vi "Create Sections from Path.vi"(8 "error in":errorcluster, 10 "Path":string, 11 "Device BaseNodeType in":T1) -> (0 "error out":errorcluster, 1 "SectionRef":T1, 2 "NewRef?":bool, 3 "Device BaseNodeType out":T1, 4 "ChannelName":string)   [LabVIEW 2010, in "RefMem PtByPt Custom Device.lvlib"]
uses:
  Custom Device/RefMem PtByPt Custom Device.lvlib
  <vilib>/NI Veristand/Custom Device API/Custom Device Pointer.ctl
  NationalInstruments.VeriStand.SystemStorage
  Custom Device/Controls/Global.vi
  <vilib>/NI Veristand/Custom Device API/Custom Device API.lvlib
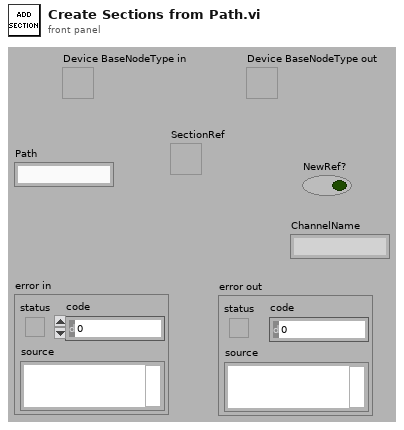
[diagram p1: front panel]
types:
  T1 = typedef "Custom Device API.lvlib/Custom Device Pointer.ctl" = refnum<k24>
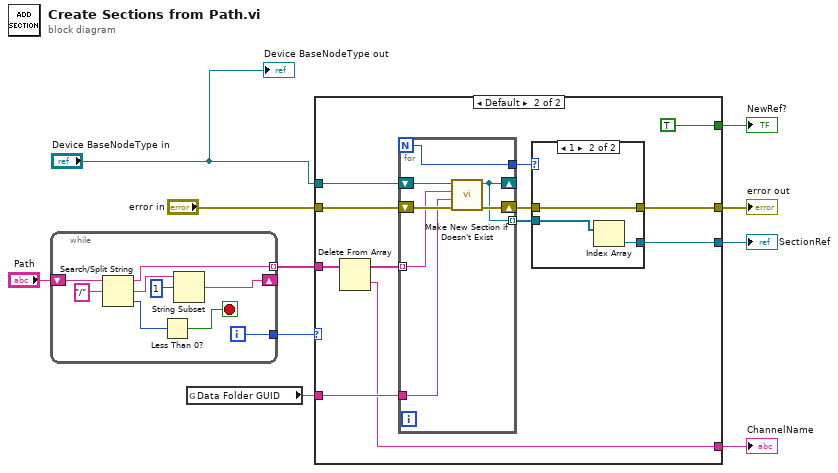
[diagram p0: block diagram]
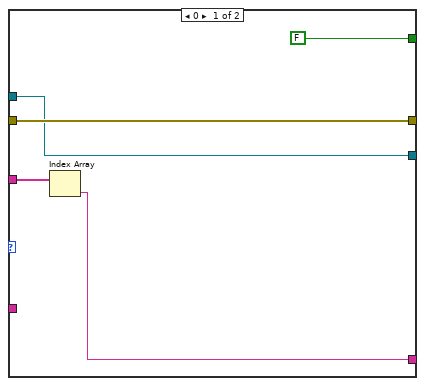
[diagram p2: hidden frame]
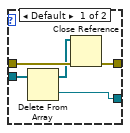
[diagram p3: hidden frame]
diagram:
  n1 = while {
    tunnel: [w15] -> w7 mode=indexing
    shift-right: [w13] -> _
    shift-left: "Path" -> [w19]
    tunnel: [w11] -> w6
    i -> [w11]
    stop <- w16 stop-if-true
    n2 = Search/Split String(string=w19, search string/char (-)="/") -> (substring before match=w15:string, match + rest of string=w14:string, offset of match=w17:i32)  [unwired: 1 in]
    n3 = Less Than 0?(x=w17) -> (x < 0?=w16:bool)
    n4 = String Subset(string=w14, offset (0)=1) -> (substring=w13:string)  [unwired: 1 in]
  }
  n5 = global read "Global.vi" "Data Folder GUID"() -> (w4:string)
  n6 = case shown="Default" w6 {
    tunnel: [w24 w29] -> w8
    tunnel: "error in" -> [w24 w35]
    tunnel: w7 -> [w22 w36]
    tunnel: "Device BaseNodeType in" -> [w20 w25]
    tunnel: w4 -> [_ w33]
    tunnel: [w20 w28] -> w3
    tunnel: [FALSE TRUE] -> w10
    tunnel: [w21 w26] -> w9
    frame 0 {
      n7 = Index Array(array=w22) -> (element=w21:string)  [unwired: 1 in]
    }
    frame Default {
      n8 = Delete From Array(array=w36) -> (deleted portion=w26:string, array with subset deleted=w34:string[])  [unwired: 2 in]
      n9 = for {
        N -> [w50]
        shift-right: [w51] -> w30
        shift-left: w35 -> [w48]
        shift-right: [w45] -> _
        shift-left: w25 -> [w49]
        tunnel: w34 -> [w47] mode=indexing
        tunnel: w33 -> [w46]
        tunnel: [w45] -> w31 mode=indexing
        tunnel: [w50] -> w32
        n10 = call "Make New Section if Doesn't Exist.vi"("error in"=w48, "Data Folder GUID"=w46, "Section Name"=w47, "Parent Section"=w49) -> ("error out"=w51:errorcluster, "New Section"=w45:refnum<k24>)  [unwired: 6 in]
      }
      n11 = case shown="1" w32 {
        tunnel: w31 -> [w41 w44]
        tunnel: [w38 w43] -> w28
        tunnel: w30 -> [w40 w42]
        tunnel: [w37 w42] -> w29
        frame Default {
          n12 = Delete From Array(array=w41) -> (deleted portion=w38:refnum<k24>, array with subset deleted=w39:refnum<k24>[])  [unwired: 2 in]
          n13 = Close Reference(reference=w39, error in (no error)=w40) -> (error out=w37:errorcluster)
        }
        frame 1 {
          n14 = Index Array(array=w44) -> (element=w43:refnum<k24>)  [unwired: 1 in]
        }
      }
    }
  }
  "NewRef?" <- w10
  "ChannelName" <- w9
  "error out" <- w8
  "SectionRef" <- w3
  "Device BaseNodeType out" <- "Device BaseNodeType in"
